vi "20TVTI_Queue_Commands.vi"(1 "VTI Control":T1, 2 "Last Status":T1, 3 "20TVTI Queue":refnum<queue>) -> (0 "New Status":T1)   [LabVIEW 2018]
uses:
  Gustav/20TVTI_Control.ctl
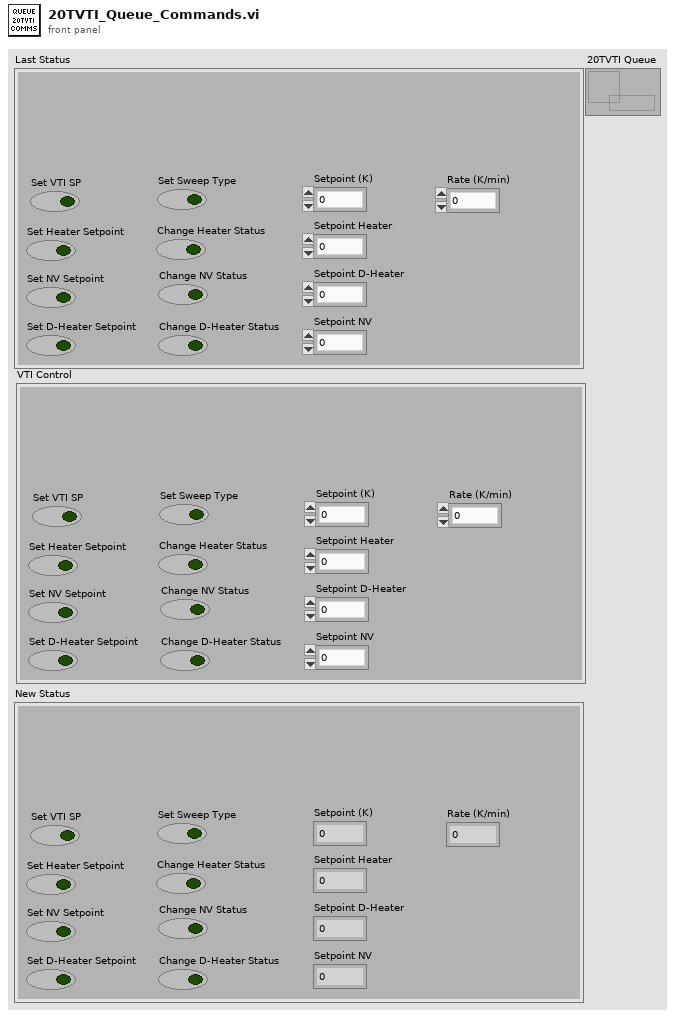
[diagram p1: front panel]
types:
  T1 = typedef "20TVTI_Control.ctl" = cluster{"Set VTI SP":bool, "Change NV Status":bool, "Set NV Setpoint":bool, "Change Heater Status":bool, "Set D-Heater Setpoint":bool, "Set Heater Setpoint":bool, "Change D-Heater Status":bool, "Set Sweep Type":bool, "Setpoint (K)":dbl, "Rate (K/min)":dbl, "Setpoint Heater":dbl, "Setpoint D-Heater":dbl, "Setpoint NV":dbl}
  T2 = cluster{"Set VTI SP":bool, "Change NV Status":bool, "Set NV Setpoint":bool, "Change Heater Status":bool, "Set D-Heater Setpoint":bool, "Set Heater Setpoint":bool, "Change D-Heater Status":bool, "Set Sweep Type":bool, "Setpoint (K)":bool, "Rate (K/min)":bool, "Setpoint Heater":bool, "Setpoint D-Heater":bool, "Setpoint NV":bool}
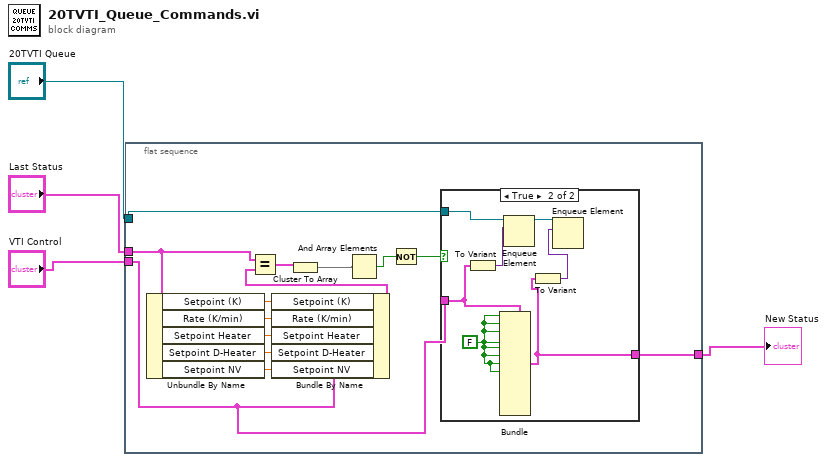
[diagram p0: block diagram]
diagram:
  n1 = flat-sequence {
    tunnel: "20TVTI Queue" -> [w18]
    tunnel: "VTI Control" -> [w12]
    tunnel: "Last Status" -> [w10]
    tunnel: [w13] -> w1
    frame #0 {
      n2 = Unbundle By Name(w10) -> ("Setpoint (K)"=w9:dbl, "Rate (K/min)"=w8:dbl, "Setpoint Heater"=w7:dbl, "Setpoint D-Heater"=w6:dbl, "Setpoint NV"=w5:dbl)
      n3 = Bundle By Name(cluster=w12, "Setpoint (K)"=w9, "Rate (K/min)"=w8, "Setpoint Heater"=w7, "Setpoint D-Heater"=w6, "Setpoint NV"=w5) -> (w11:T1)
      n4 = Equal?(x=w10, y=w11) -> (x = y?=w14:T2)
      n5 = Cluster To Array(cluster=w14) -> (array=w17:bool[])
      n6 = And Array Elements(Boolean array=w17) -> (logical AND=w16:bool)
      n7 = Not(x=w16) -> (.not. x?=w15:bool)
      n8 = case shown="True" w15 {
        tunnel: w18 -> [_ w26]
        tunnel: w12 -> [w19 w22]
        tunnel: [w19 w20] -> w13
        frame False {
        }
        frame True {
          w21 = FALSE
          n9 = To Variant(anything=w22) -> (Variant=w25:variant)
          n10 = Bundle(cluster=w22, "Set VTI SP"=w21, "Change NV Status"=w21, "Set NV Setpoint"=w21, "Change Heater Status"=w21, "Set D-Heater Setpoint"=w21, "Set Heater Setpoint"=w21, "Change D-Heater Status"=w21, "Set Sweep Type"=w21) -> (w20:T1)  [unwired: 5 in]
          n11 = Enqueue Element(queue=w26, element=w25) -> (queue out=w24:refnum<queue>)  [unwired: 2 in, 2 out]
          n12 = To Variant(anything=w20) -> (Variant=w23:variant)
          n13 = Enqueue Element(queue=w24, element=w23) -> ()  [unwired: 2 in, 3 out]
        }
      }
    }
  }
  "New Status" <- w1
